vi "user interface.vi"() -> ()   [LabVIEW 2018]
uses:
  <vilib>/Tufts CEEO ROS for LabVIEW Software/ROS/Code/SubVIs/_ROSControl.ctl
  <vilib>/Tufts CEEO ROS for LabVIEW Software/ROS/Code/SubVIs/_ROSDirection.ctl
  <vilib>/Tufts CEEO ROS for LabVIEW Software/ROS/Code/Console/Servers/ServerSubs/TopicDef.ctl
  <vilib>/Tufts CEEO ROS for LabVIEW Software/ROS/MessageBuilding/std_msgs/subs/stringScalar.vi
panel:
  in  "stop":bool
  in  "Start Scanning":bool
  in  "stop Scan":bool
  in  "Start Registring the Robot Position":bool
  out "Scan Details":T1={"Min. Angle (rad)"=-2.3561899662017822, "Max. Angle (rad)"=2.3561899662017822, "Angle Incr. (rad)"=0.006554075051099062, "Time Inc. (s)"=0.0, "Scan Time (s)"=0.0, "Min. Range (m)"=0.10000000149011612, "Max. Range (m)"=1.0089348943138683e-42}
  out "Laser Scan Plot (in Husky Frame)":cluster{dbl[], dbl[]}(graph)
  out "Array":cluster{"x":dbl, "y":dbl}[](array[cluster])
  out "Odom Error Out":errorcluster
  out "Scan Error Out":errorcluster
  in  "Stop Position":bool
  out "Husky Pose Plot":cluster{"X":dbl, "Y":dbl}[](graph)=[{"X"=2.1588546690121686, "Y"=0.6824320147682317}]
  out "Husky EKF Odometry":T2={"PoseCovariance"={"Pose"={"Position\n(xyz)"={"x"=2.1588546690121686, "y"=0.6824320147682317, "z"=0.0}, "Orientation\n(Quaternions)"={"x"=0.0, "y"=0.0, "z"=-0.6154075833582808, "w"=0.7882090499005455}}, "Covariance[1,1]"=150.49515067805697}}
  out "2D Pose":cluster{"x":dbl, "y":dbl}={"x"=2.1588546690121686, "y"=0.6824320147682317}
  in  "Update Time (ms)":u32=300
  in  "Clear Plot":bool
  in  "Max Odom Pts":dbl=500.0
  in  "Manual/\nAUTONOMOUS":bool
  out "ROS out":T3={"topic port"=0, "Node"="", "topic"="", "type"="", "node port"=0, "error "={"status"=FALSE, "code"=0, "source"=""}, "Direction"=enum."Node", "Update (ms)"=1, "FIFO size"=1}
  in  "DOWN":bool
  in  "TOP":bool
  in  "RIGHT":bool
  in  "LEFT":bool
  in  "STOP Manual mode":bool
  in  "THETA POSITION":dbl
  in  "X POSITION":dbl
  out "ROBOT SPEED":dbl(knob) scale=0.0..10.0
  out "error out":errorcluster
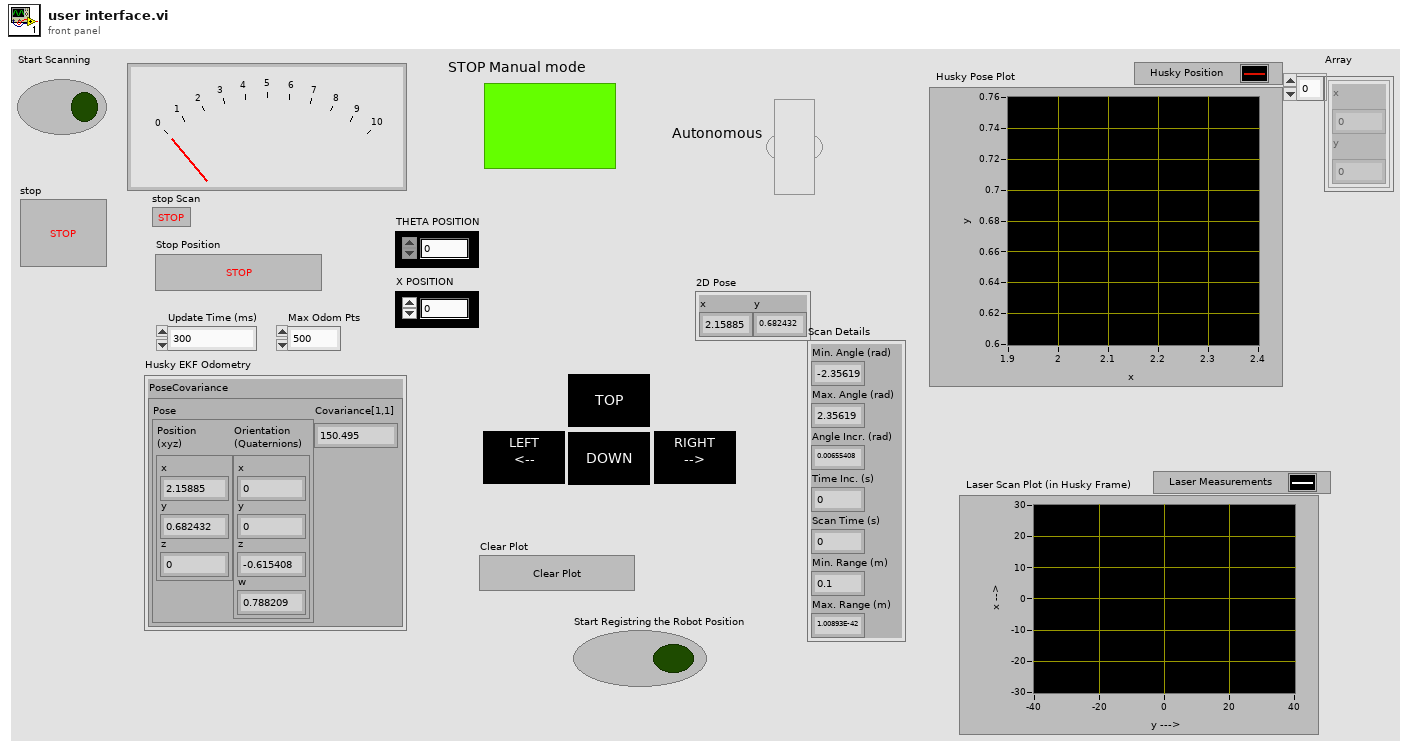
[diagram p1: front panel]
types:
  T1 = cluster{"Min. Angle (rad)":dbl, "Max. Angle (rad)":dbl, "Angle Incr. (rad)":dbl, "Time Inc. (s)":dbl, "Scan Time (s)":dbl, "Min. Range (m)":dbl, "Max. Range (m)":dbl}
  T2 = cluster{"PoseCovariance":cluster{"Pose":cluster{"Position\n(xyz)":cluster{"x":dbl, "y":dbl, "z":dbl}, "Orientation\n(Quaternions)":cluster{"x":dbl, "y":dbl, "z":dbl, "w":dbl}}, "Covariance[1,1]":dbl}}
  T3 = typedef "_ROSControl.ctl" = cluster{"topic port":u16, "Node":string, "topic":string, "type":string, "node port":u16, "error ":errorcluster, "Direction":T4, "Update (ms)":u16, "FIFO size":u16}
  T4 = typedef "_ROSDirection.ctl" = enum16{"Node", "Publisher", "Subscriber", "ServiceClient", "ServiceProvider"}
  T5 = typedef "TopicDef.ctl" = cluster{"Topic":string, "Type":string, "Action":T4, "Update (ms)":u16, "queue size":u16}
  T6 = cluster{"PoseCovariance":cluster{"Pose":cluster{"Point":cluster{"x":dbl, "y":dbl, "z":dbl}, "Quaternion":cluster{"x":dbl, "y":dbl, "z":dbl, "w":dbl}}, "Covariance":dbl}}
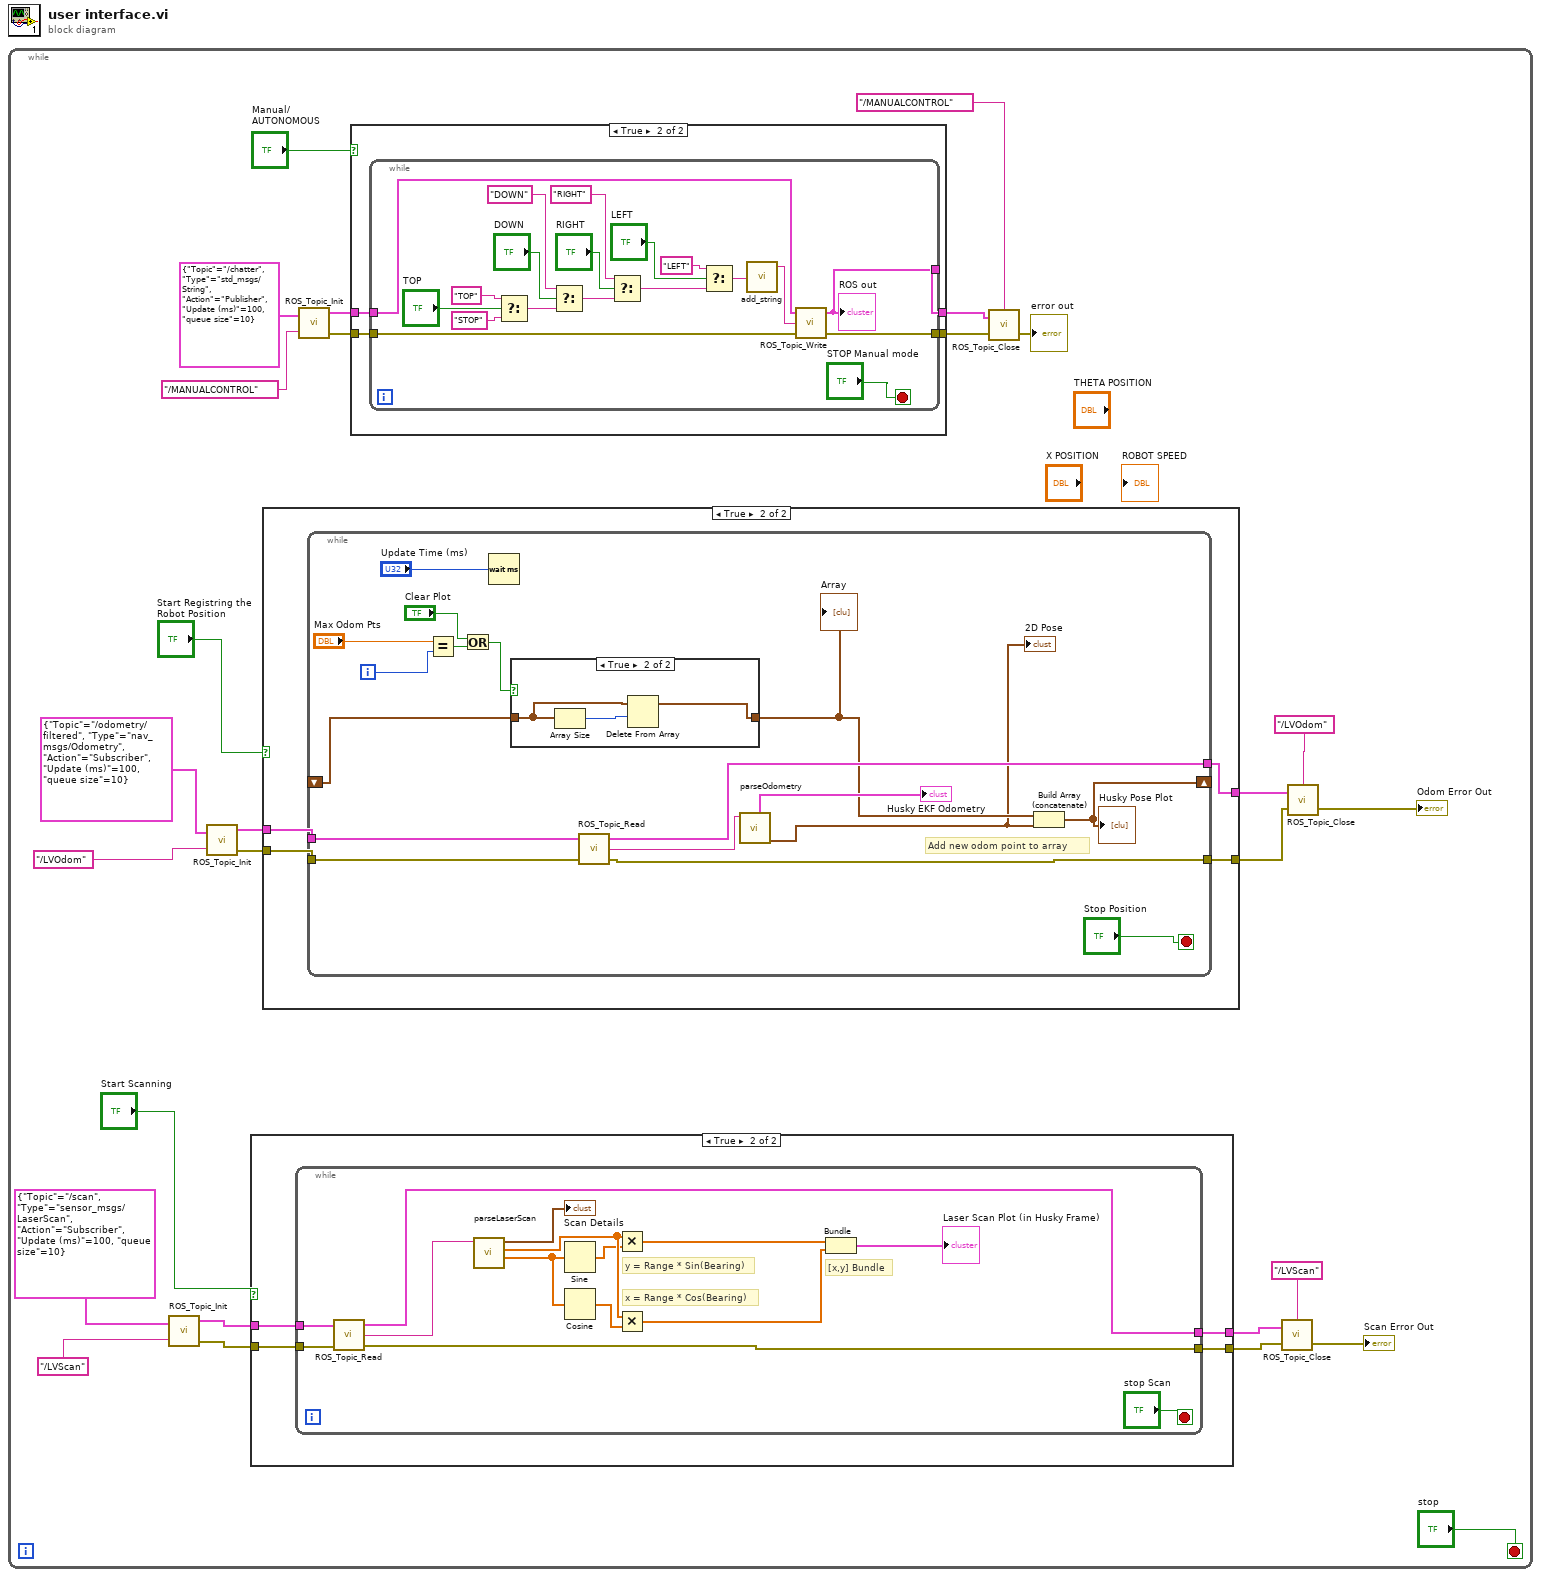
[diagram p0: block diagram]
diagram:
  n1 = while {
    stop <- "stop" stop-if-true
    n2 = call <vilib>:"ROS_Topic_Init.vi"("Definitions"=T5 {"Topic"="/scan", "Type"="sensor_msgs/LaserScan", "Action"=enum."Subscriber", "Update (ms)"=100, "queue size"=10}, "node"="/LVScan") -> ("ROS out"=w7:T3, "error out"=w6:errorcluster)  [unwired: 1 in]
    n3 = call <vilib>:"ROS_Topic_Init.vi"("Definitions"=T5 {"Topic"="/odometry/filtered", "Type"="nav_msgs/Odometry", "Action"=enum."Subscriber", "Update (ms)"=100, "queue size"=10}, "node"="/LVOdom") -> ("ROS out"=w15:T3, "error out"=w14:errorcluster)  [unwired: 1 in]
    n4 = case shown="True" "Start Scanning" {
      tunnel: [w30 w34] -> w9
      tunnel: [w29 w33] -> w8
      tunnel: w7 -> [w30 w32]
      tunnel: w6 -> [w29 w31]
      frame False {
      }
      frame True {
        n5 = while {
          tunnel: [w39] -> w34
          tunnel: [w38] -> w33
          tunnel: w32 -> [w37]
          tunnel: w31 -> [w36]
          stop <- "stop Scan" stop-if-true
          # "[x,y] Bundle"
          # "y = Range * Sin(Bearing)"
          # "x = Range * Cos(Bearing)"
          n6 = call <vilib>:"ROS_Topic_Read.vi"("error in (no error)"=w36, "ROS in"=w37) -> ("error out"=w38:errorcluster, "Reply"=w48:string, "ROS out"=w39:T3)  [unwired: 1 in]
          n7 = call "parseLaserScan.vi"("msg in"=w48) -> ("Bearing Array"=w46:dbl[], "Range Array"=w45:sgl[], "Scan Details"=→"Scan Details":T1)  [unwired: 3 in, 1 out]
          n8 = Sine(x=w46) -> (sin(x)=w44:dbl[])
          n9 = Cosine(x=w46) -> (cos(x)=w47:dbl[])
          n10 = Multiply(x=w45, y=w44) -> (x*y=w41:dbl[])
          n11 = Multiply(x=w45, y=w47) -> (x*y=w42:dbl[])
          n12 = Bundle(w41, w42) -> (→"Laser Scan Plot (in Husky Frame)":cluster{dbl[], dbl[]})  [unwired: 1 in]
        }
      }
    }
    n13 = case shown="True" "Start Registring the Robot Position" {
      tunnel: w15 -> [w50 w54]
      tunnel: w14 -> [w49 w53]
      tunnel: [w50 w52] -> w5
      tunnel: [w49 w51] -> w4
      frame False {
      }
      frame True {
        n14 = while {
          shift-right: [w70] -> _
          shift-left: _ -> [w57]
          tunnel: w54 -> [w67]
          tunnel: w53 -> [w66]
          tunnel: [w64] -> w52
          tunnel: [w63] -> w51
          i -> [w60]
          stop <- "Stop Position" stop-if-true
          # "Add new odom point to array"
          n15 = Equal?(x="Max Odom Pts", y=w60) -> (x = y?=w59:bool)
          n16 = Or(x="Clear Plot", y=w59) -> (x .or. y?=w58:bool)
          n17 = Wait (ms)(milliseconds to wait="Update Time (ms)") -> ()  [unwired: 1 out]
          n18 = case shown="True" w58 {
            tunnel: [w72 w74] -> w56
            tunnel: w57 -> [w72 w73]
            frame False {
            }
            frame True {
              n19 = Array Size(array=w73) -> (size(s)=w75:i32)
              n20 = Delete From Array "Delete From Array"(array=w73, length=w75) -> (array with subset deleted=w74:cluster{"x":dbl, "y":dbl}[])  [unwired: 1 in, 1 out]
            }
          }
          "Array" <- w56
          n21 = call <vilib>:"ROS_Topic_Read.vi"("error in (no error)"=w66, "ROS in"=w67) -> ("error out"=w63:errorcluster, "Reply"=w69:string, "ROS out"=w64:T3)  [unwired: 1 in]
          n22 = call "parseOdometry.vi"("msg in"=w69) -> ("Odometry"=→"Husky EKF Odometry":T6, "Pose 2D"=w55:cluster{"x":dbl, "y":dbl})  [unwired: 3 in, 3 out]
          "2D Pose" <- w55
          n23 = Build Array (concatenate)(w56, w55) -> (w70:cluster{"x":dbl, "y":dbl}[])
          "Husky Pose Plot" <- w70
        }
      }
    }
    n24 = call <vilib>:"ROS_Topic_Init.vi"("Definitions"=T5 {"Topic"="/chatter", "Type"="std_msgs/String", "Action"=enum."Publisher", "Update (ms)"=100, "queue size"=10}, "node"="/MANUALCONTROL") -> ("ROS out"=w21:T3, "error out"=w28:errorcluster)  [unwired: 1 in]
    n25 = case shown="True" "Manual/\nAUTONOMOUS" {
      tunnel: w28 -> [w76 w78]
      tunnel: w21 -> [w77 w79]
      tunnel: [w77 w80] -> w23
      tunnel: [w76 w81] -> w22
      frame False {
      }
      frame True {
        n26 = while {
          tunnel: w79 -> [w91]
          tunnel: [w99] -> w80
          tunnel: w78 -> [w90]
          tunnel: [w100] -> w81
          stop <- "STOP Manual mode" stop-if-true
          n27 = Select(t="TOP", s="TOP", f="STOP") -> (s? t:f=w98:string)
          n28 = Select(t="DOWN", s="DOWN", f=w98) -> (s? t:f=w97:string)
          n29 = Select(t="RIGHT", s="RIGHT", f=w97) -> (s? t:f=w87:string)
          n30 = Select(t="LEFT", s="LEFT", f=w87) -> (s? t:f=w84:string)
          n31 = call-poly <vilib>:"add_string.vi"("String"=w84) -> ("msg out"=w83:string)  [unwired: 4 in]
          n32 = call <vilib>:"ROS_Topic_Write.vi"("error in (no error)"=w90, "Msg in"=w83, "ROS in"=w91) -> ("error out"=w100:errorcluster, "ROS out"=w99:T3)  [unwired: 1 in]
          "ROS out" <- w99
        }
      }
    }
    n33 = call <vilib>:"ROS_Topic_Close.vi"("error in"=w22, "ROS in"=w23, "node"="/MANUALCONTROL") -> ("error out"=→"error out":errorcluster)  [unwired: 1 in]
    n34 = call <vilib>:"ROS_Topic_Close.vi"("error in"=w8, "ROS in"=w9, "node"="/LVScan") -> ("error out"=→"Scan Error Out":errorcluster)  [unwired: 1 in]
    n35 = call <vilib>:"ROS_Topic_Close.vi"("error in"=w4, "ROS in"=w5, "node"="/LVOdom") -> ("error out"=→"Odom Error Out":errorcluster)  [unwired: 1 in]
  }
